vi "Time Stamp To String.vi"(1 "Time Stamp":timestamp) -> (0 "Output string":string)   [LabVIEW 2023, in "Utilities.lvlib"]
uses:
  Utilities.lvlib
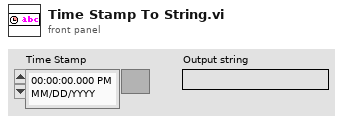
[diagram p1: front panel]
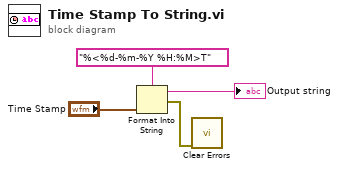
[diagram p0: block diagram]
diagram:
  n1 = Format Into String(format string="%<%d-%m-%Y %H:%M>T", "Time Stamp") -> (resulting string=→"Output string":string, error out=w3:errorcluster)  [unwired: 2 in]
  n2 = call <vilib>:"Clear Errors.vi"("error in (no error)"=w3) -> ()  [unwired: 5 in, 2 out]
